vi "StoneColor.vi"(8 "error in (no error)":errorcluster, 11 "Player in":refnum<class "Player.lvclass">) -> (0 "error out":errorcluster, 2 "StoneColor":u16, 3 "Player out":refnum<class "Player.lvclass">)   [LabVIEW 2009, in "Player.lvclass"]
doc: "Get the Stone Color of the current player"
uses:
  Player.lvclass
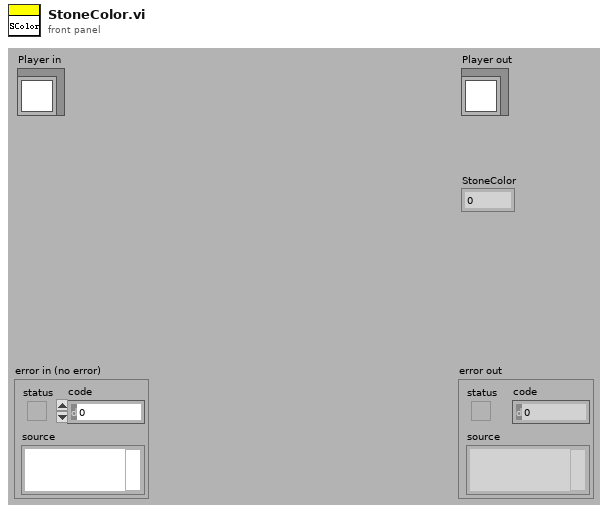
[diagram p1: front panel]
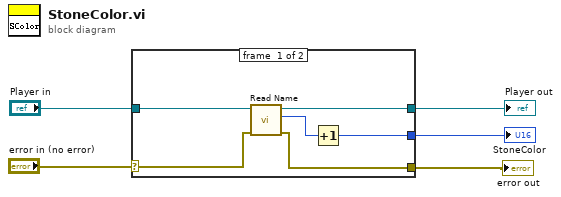
[diagram p0: block diagram]
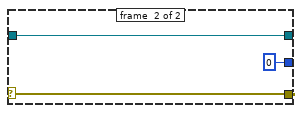
[diagram p2: hidden frame]
diagram:
  n1 = case shown="No Error" "error in (no error)" {
    selector: "error in (no error)" -> [w9 w14]
    tunnel: [w8 w14] -> w4
    tunnel: [w10 w13] -> w2
    tunnel: "Player in" -> [w11 w13]
    tunnel: [w6 u16 0] -> w1
    frame #0 {
      n2 = call "Read Name.vi"("error in (no error)"=w9, "Player in"=w11) -> ("error out"=w8:errorcluster, "Name"=w7:u16, "Player out"=w10:refnum<class "Player.lvclass">)  [unwired: 7 in]
      n3 = Increment(x=w7) -> (x+1=w6:u16)
    }
    frame #1 {
    }
  }
  "error out" <- w4
  "Player out" <- w2
  "StoneColor" <- w1
